vi "StateToColor.vi"(8 "error in (no error)":errorcluster, 11 "Flags in":refnum<class "Flags.lvclass">) -> (0 "error out":errorcluster, 2 "RoomNumFlags":T1={"Room Number"=0, "Flag State"=[1, 3, 5, 7]}, 3 "Flags out":refnum<class "Flags.lvclass">)   [LabVIEW 2015, in "Flags.lvclass"]
uses:
  Flags.lvclass
  TypeDef/ColorFlags.ctl
  Flags.lvclass/Flags.ctl
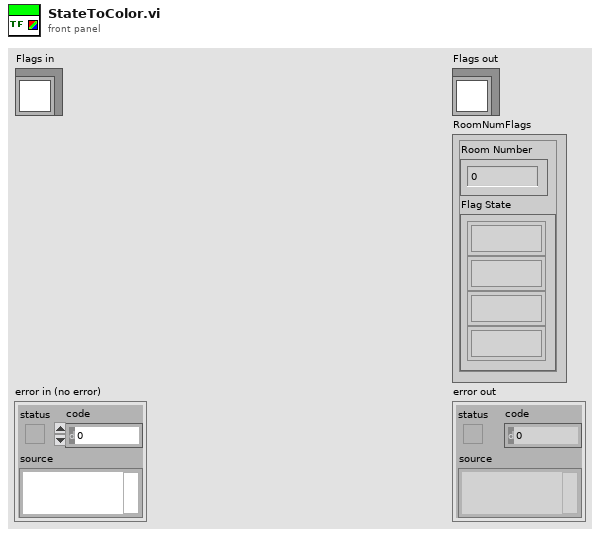
[diagram p1: front panel]
types:
  T1 = typedef "ColorFlags.ctl" = cluster{"Room Number":u32, "Flag State":u8[]}
  T2 = typedef "Flags.lvclass/ColorEnum.ctl" = enum8{"Red", "Blue", "Green", "Yellow"}
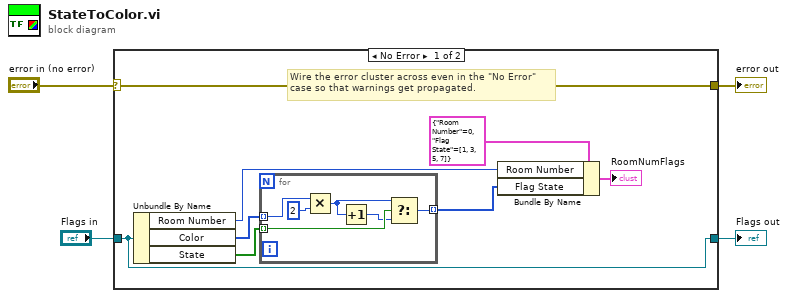
[diagram p0: block diagram]
diagram:
  n1 = case shown="No Error" "error in (no error)" {
    selector: "error in (no error)" -> [w12 w20]
    tunnel: [w12 w20] -> w3
    tunnel: [w11 w19] -> w1
    tunnel: "Flags in" -> [w11 w19]
    frame No Error {
      # "Wire the error cluster across even in the \"No Error\"\ncase so that warnings get propagated."
      n2 = Unbundle By Name(w11) -> ("Room Number"=w6:u32, "Color"=w10:T2[], "State"=w9:bool[])
      n3 = for {
        tunnel: w10 -> [w16] mode=indexing
        tunnel: w9 -> [w17] mode=indexing
        tunnel: [w13] -> w5 mode=indexing
        n4 = Multiply(x=w16, y=u8 2) -> (x*y=w14:u8)
        n5 = Increment(x=w14) -> (x+1=w15:u8)
        n6 = Select(t=w14, s=w17, f=w15) -> (s? t:f=w13:u8)
      }
      n7 = Bundle By Name(cluster=T1 {"Room Number"=0, "Flag State"=[1, 3, 5, 7]} ("Array"), "Room Number"=w6, "Flag State"=w5) -> (→"RoomNumFlags":T1)
    }
    frame Error {
    }
  }
  "error out" <- w3
  "Flags out" <- w1
